vi "server api address.vi"() -> (3 "Server API URL":string)   [LabVIEW 2024]
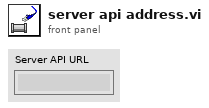
[diagram p1: front panel]
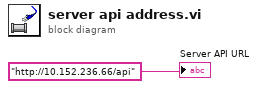
[diagram p0: block diagram]
diagram:
  "Server API URL" <- "http://10.152.236.66/api" ("Server API URL")
